vi "PANEL.vi"() -> ()   [LabVIEW 2021]
panel:
  out "Waveform Chart":dbl(graph)
  in  "Slide":dbl(slide) scale=0.0..10.0
  in  "Stop":bool
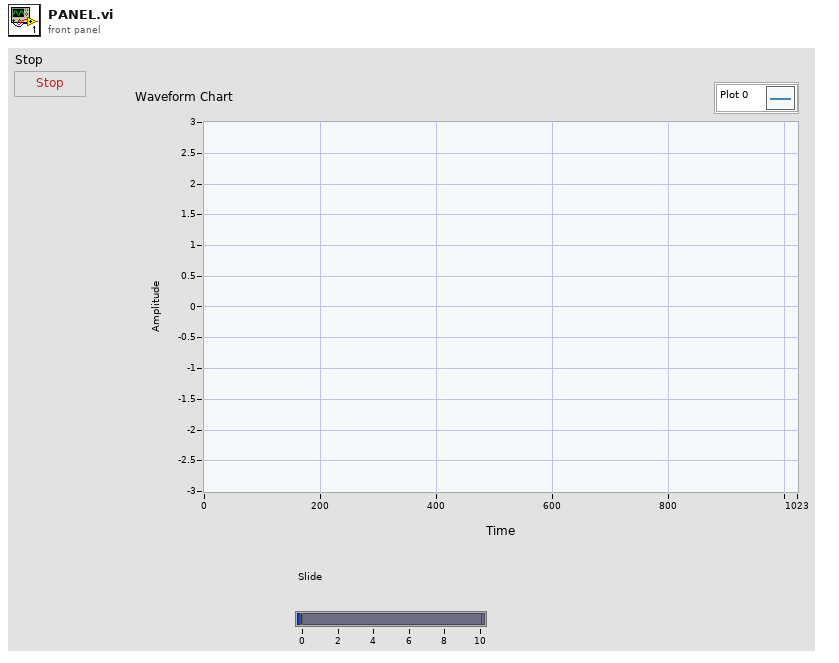
[diagram p1: front panel]
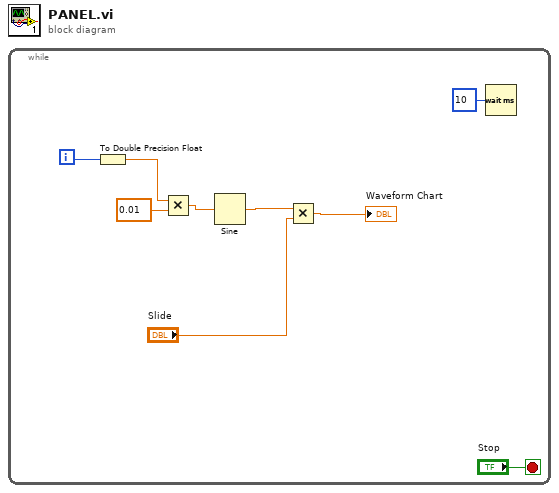
[diagram p0: block diagram]
diagram:
  n1 = while {
    i -> [w3]
    stop <- "Stop" stop-if-true
    n2 = To Double Precision Float(number=w3) -> (double precision float=w4:dbl)
    n3 = Multiply(x=w4, y=0.01) -> (x*y=w7:dbl)
    n4 = Sine(x=w7) -> (sin(x)=w6:dbl)
    n5 = Multiply(x=w6, y="Slide") -> (x*y=→"Waveform Chart":dbl)
    n6 = Wait (ms)(milliseconds to wait=u32 10) -> ()  [unwired: 1 out]
  }
